vi "AboutCamera.vi"() -> ()   [LabVIEW 2015]
uses:
  <vilib>/vision/driver/IMAQdx.llb/IMAQdx Attribute Visibility.ctl
  <vilib>/vision/driver/IMAQdx.llb/IMAQdx Attribute Type.ctl
  <vilib>/vision/driver/NI_Vision_Acquisition_Software.lvlib
panel:
  out "Current Mode":u32
  out "Video Modes":T1(array[cluster])
  out "Attribute Information Array":T3(array[cluster])
  in  "Root":string
  in  "Visibility":T4=enum."Advanced"
  out "Camera Information Array":T5(array[cluster]) {"BusType" format="%x"; "SerialNumberLow" format="%.0x"; "SerialNumberHigh" format="%.0x"}
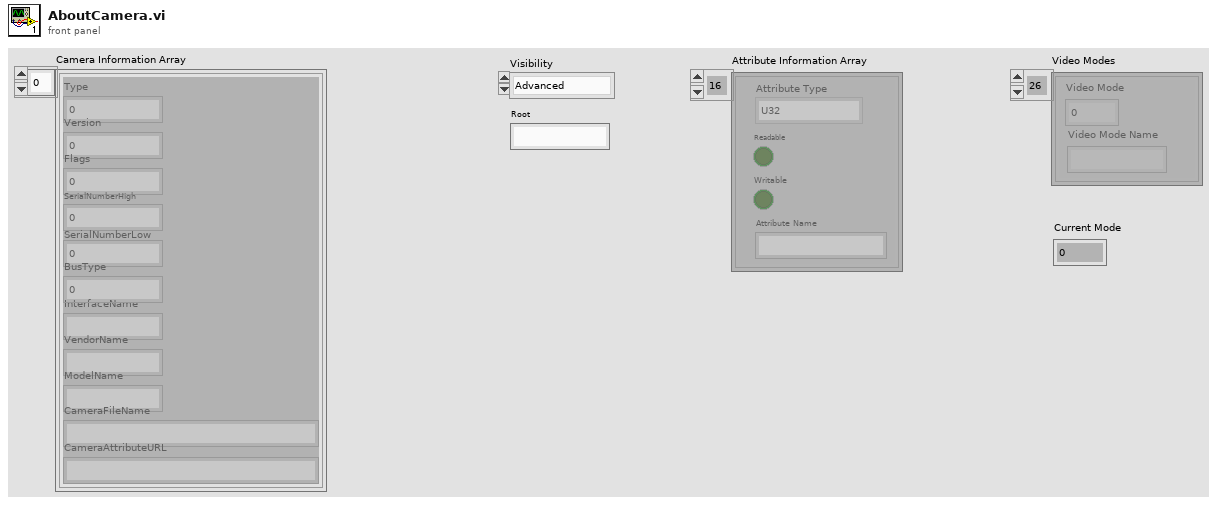
[diagram p1: front panel]
types:
  T1 = cluster{"Video Mode":u32, "Video Mode Name":string}[]
  T2 = typedef "NI_Vision_Acquisition_Software.lvlib/IMAQdx Attribute Type.ctl" = enum32{"U32", "I64", "DBL", "String", "Enum", "Bool", "Command"}
  T3 = cluster{"Attribute Type":T2, "Readable":bool, "Writable":bool, "Attribute Name":string}[]
  T4 = typedef "NI_Vision_Acquisition_Software.lvlib/IMAQdx Attribute Visibility.ctl" = enum32{"Simple", "Intermediate", "Advanced"}
  T5 = cluster{"Type":u32, "Version":u32, "Flags":u32, "SerialNumberHigh":u32, "SerialNumberLow":u32, "BusType":u32, "InterfaceName":string, "VendorName":string, "ModelName":string, "CameraFileName":string, "CameraAttributeURL":string}[]
  T6 = cluster{"Type":u32, "Version":u32, "Flags":u32, "SerialNumberHigh":u32, "SerialNumberLow":u32, "BusType":u32, "InterfaceName":string, "VendorName":string, "ModelName":string, "CameraFileName":string, "CameraAttributeURL":string}
  T7 = typedef "IMAQdx.ctl" = refnum<k21>
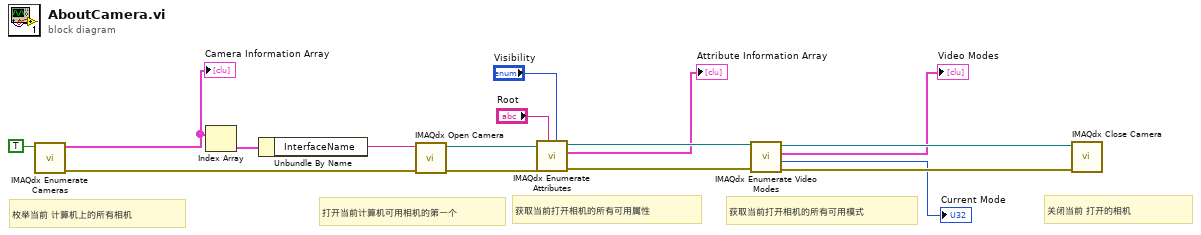
[diagram p0: block diagram]
diagram:
  # "关闭当前 打开的相机"
  # "获取当前打开相机的所有可用模式"
  # "获取当前打开相机的所有可用属性"
  # "打开当前计算机可用相机的第一个"
  # "枚举当前 计算机上的所有相机"
  n1 = call <vilib>:"IMAQdx Enumerate Cameras.vi"("Connected Only? (Yes)"=TRUE) -> ("error out"=w12:errorcluster, "Camera Information Array"=w15:T5)  [unwired: 9 in]
  "Camera Information Array" <- w15
  n2 = Index Array(array=w15) -> (element=w14:T6)  [unwired: 1 in]
  n3 = Unbundle By Name(w14) -> ("InterfaceName"=w13:string)
  n4 = call <vilib>:"IMAQdx Open Camera.vi"("error in"=w12, "Session In"=w13) -> ("error out"=w10:errorcluster, "Session Out"=w11:T7)  [unwired: 8 in]
  n5 = call <vilib>:"IMAQdx Enumerate Attributes.vi"("Visibility"="Visibility", "Root"="Root", "error in"=w10, "Session In"=w11) -> ("error out"=w6:errorcluster, "Attribute Information Array"=→"Attribute Information Array":T3, "Session Out"=w7:T7)  [unwired: 5 in]
  n6 = call <vilib>:"IMAQdx Enumerate Video Modes.vi"("error in"=w6, "Session In"=w7) -> ("error out"=w4:errorcluster, "Current Mode"=→"Current Mode":u32, "Video Modes"=→"Video Modes":T1, "Session Out"=w5:T7)  [unwired: 6 in]
  n7 = call <vilib>:"IMAQdx Close Camera.vi"("error in"=w4, "Session In"=w5) -> ()  [unwired: 9 in, 1 out]
